vi "Example_eCompassCompensation.vi"   [LabVIEW 2023]
uses:
  D:/Proj/RoboticLawnMower/Software/LabView/dotNET/eCompass.dll
  dotNET/eCompass.dll
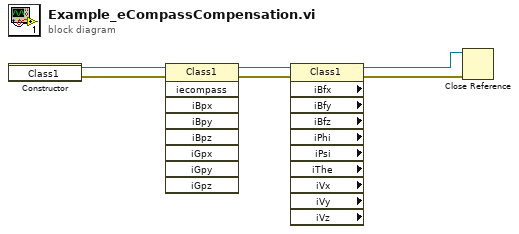
[diagram p0: block diagram]
diagram:
  n1 = constructor class="Class1"() -> (reference out=w6:refnum<k24>, error out=w5:errorcluster)  [unwired: 3 in, 1 out]
  n2 = invoke class="Class1" method="iecompass"(reference=w6, error in=w5) -> (reference out=w4:refnum<k24>, error out=w3:errorcluster)  [unwired: 7 in, 7 out]
  n3 = property class="Class1" props=["iBfx", "iBfy", "iBfz", "iPhi", "iPsi", "iThe", "iVx", "iVy", "iVz"](reference=w4, error in=w3) -> (reference out=w1:refnum<k24>, error out=w2:errorcluster)  [unwired: 9 out]
  n4 = Close Reference(reference=w1, error in (no error)=w2) -> ()  [unwired: 1 out]
